vi "XIPIN_AXI_Memory_Mapped_to_Stream_Mapper_1_1.vi"   [LabVIEW 2017]
doc: "The AXI Memory Mapped to Stream Mapper.\n------------------------------------\n<b>Need License</b> : No\n<b>Interface</b> : AXI4 AXI4-Stream"
uses:
  <vilib>/rvi/XilinxIP/XIPIN_XNode/niFpgaXIPIN.xnode
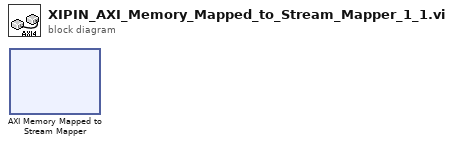
[diagram p0: block diagram]
diagram:
  n1 = xnode ("AXI Memory Mapped to Stream Mapper")() -> ()
